vi "FL_Get_TTL_in_pulse_length.vi"(1 "Reset":bool, 2 "Latest sensor input (decoded)":string[](array[string])) -> (0 "TTL pulse length, ms":u32)   [LabVIEW 2018, in "Tracker.lvlib"]
uses:
  Tracker.lvlib
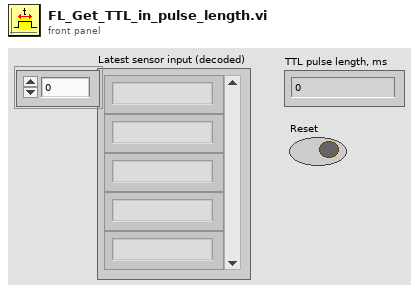
[diagram p1: front panel]
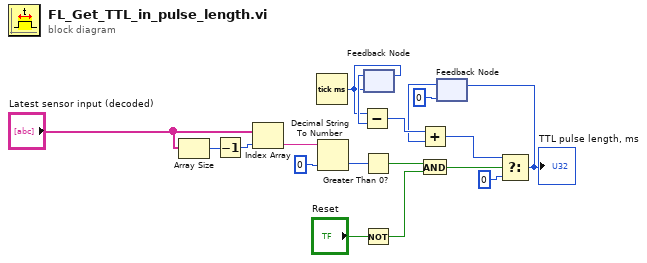
[diagram p0: block diagram]
diagram:
  n1 = Array Size(array="Latest sensor input (decoded)") -> (size(s)=w16:i32)
  n2 = Decrement(x=w16) -> (x-1=w18:i32)
  n3 = Index Array(array="Latest sensor input (decoded)", index=w18) -> (element=w15:string)
  n4 = Tick Count (ms)() -> (millisecond timer value=w1:u32)
  n5 = Decimal String To Number(string=w15, default (0L)=u8 0 ("default (0 I32)")) -> (number=w13:u8)  [unwired: 1 in, 1 out]
  n6 = Greater Than 0?(x=w13) -> (x > 0?=w12:bool)
  n7 = Not(x="Reset") -> (.not. x?=w2:bool)
  n8 = feedback #1(w1) -> (w11:u32)
  n9 = Subtract(x=w1, y=w11) -> (x-y=w10:u32)
  n10 = feedback-in #1(w1) -> ()
  n11 = And(x=w12, y=w2) -> (x .and. y?=w4:bool)
  n12 = feedback #2(u32 0) -> (w9:u32)
  n13 = Add(x=w10, y=w9) -> (x+y=w7:u32)
  n14 = Select(t=w7, s=w4, f=u32 0) -> (s? t:f=w5:u32)
  "TTL pulse length, ms" <- w5
  n15 = feedback-in #2(w5) -> ()
